vi "Get Targets IP Address info.vi"() -> (1 "IP Address":string, 2 "ID":string)   [LabVIEW 2020]
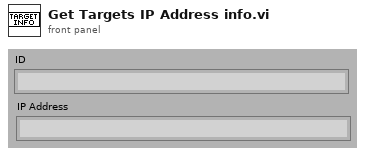
[diagram p1: front panel]
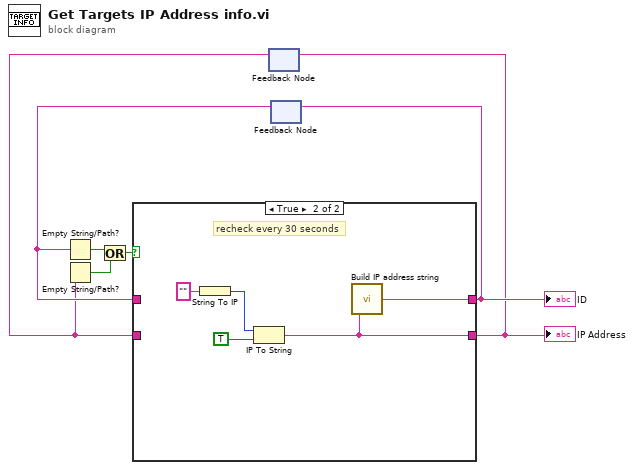
[diagram p0: block diagram]
diagram:
  n1 = feedback #1() -> (w2:string)  [unwired: 1 in]
  n2 = Empty String/Path?(string/path=w2) -> (empty?=w1:bool)
  n3 = feedback #2() -> (w3:string)  [unwired: 1 in]
  n4 = Empty String/Path?(string/path=w3) -> (empty?=w4:bool)
  n5 = Or(x=w4, y=w1) -> (x .or. y?=w5:bool)
  n6 = case shown="True" w5 {
    tunnel: [w9 w11] -> w7
    tunnel: [w8 w10] -> w6
    tunnel: w3 -> [w9 _]
    tunnel: w2 -> [w8 _]
    frame False {
    }
    frame True {
      # "recheck every 30 seconds"
      n7 = String To IP(1:"" ("name")) -> (0:w13:u32)
      n8 = IP To String(1:TRUE ("dot notation? (F)"), 2:w13) -> (0:w10:string)
      n9 = call "Build IP address string.vi"("IP address"=w10) -> ("IP Name"=w11:string)  [unwired: 4 in]
    }
  }
  "ID" <- w7
  "IP Address" <- w6
  n10 = feedback-in #1(w6) -> ()
  n11 = feedback-in #2(w7) -> ()
